vi "Reset1212(Host).vi"(2 "error in":errorcluster, 3 "FPGA Interface In":refnum<k20>) -> (0 "error out":errorcluster, 1 "FPGA Interface Out":refnum<k20>)   [LabVIEW 2018]
uses:
  <vilib>/userdefined/High Color/nirio_resource_hc.ctl
  <vilib>/FPGAPlugInAG/Dynamic/niLvFpga_Reset_Dynamic.vi
  <vilib>/Utility/error.llb/Error Cluster From Error Code.vi
  <vilib>/rvi/errors/niLvFpgaAdjustHostInterfaceError.vi
  <vilib>/FPGAPlugInAG/Dynamic/niLvFpga_Run_Dynamic.vi
  <vilib>/FPGAPlugInAG/Dynamic/niLvFpga_Close_Dynamic.vi
  <vilib>/rvi/interface/nirviMethod/nirviMethod.xnode
  <vilib>/rvi/interface/nirviReadWriteControl/nirviReadWriteControl.xnode
  <vilib>/rvi/interface/nirviCloseFPGA/nirviCloseFPGA.xnode
  NiFpgaLv.dll
  <vilib>/rvi/interface/Simulation/niFpgaSimulationCallBeginRW.vi
panel:
  in  "DEBUG":bool
  in  "resource name":T1="RIO0" caption="RIO Device"
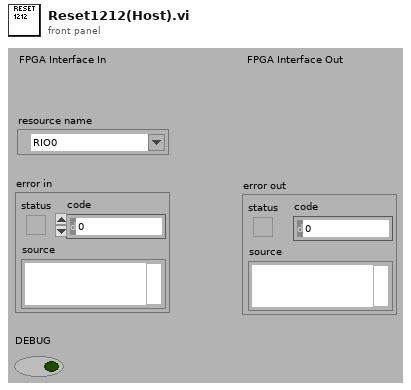
[diagram p1: front panel]
types:
  T1 = typedef "nirio_resource_hc.ctl" = tag
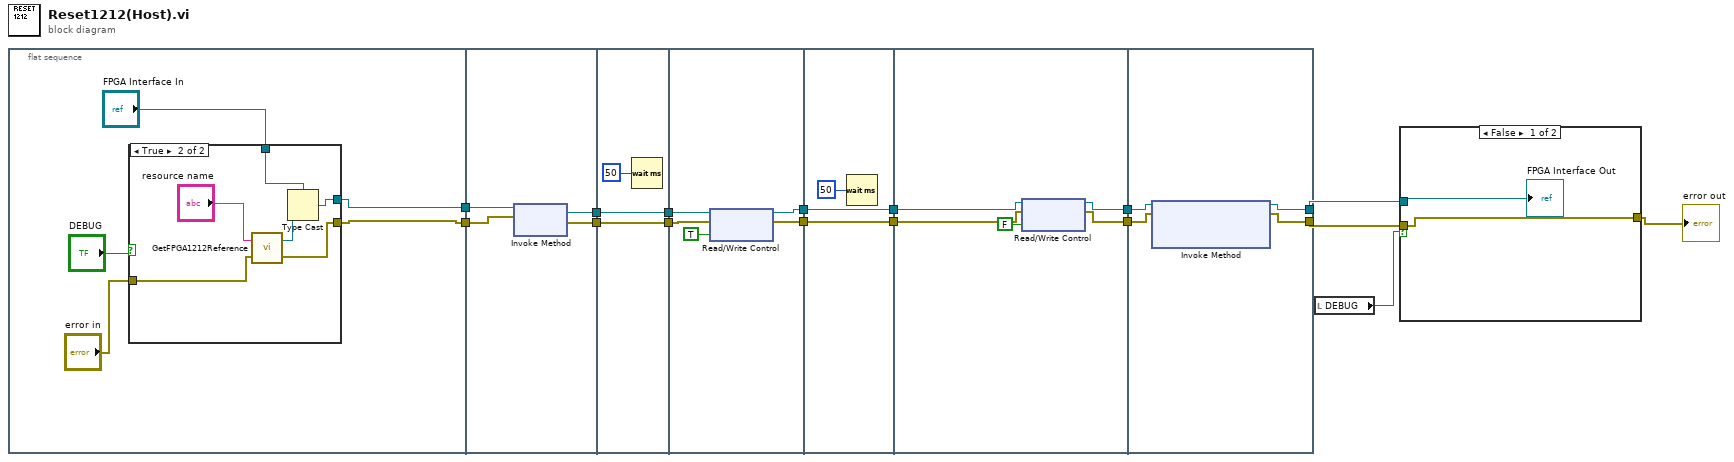
[diagram p0: block diagram]
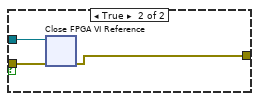
[diagram p2: hidden frame]
diagram:
  n1 = flat-sequence {
    tunnel: [w17] -> w9
    tunnel: [w18] -> w4
    tunnel: [w32] -> w8
    tunnel: w9 -> [w33]
    tunnel: [w31] -> w6
    tunnel: w4 -> [w30]
    tunnel: w8 -> [w36]
    tunnel: [w36] -> w7
    tunnel: w6 -> [w35]
    tunnel: [w35] -> w5
    tunnel: [w41] -> w16
    tunnel: [w40] -> w13
    tunnel: w7 -> [w37]
    tunnel: w5 -> [w38]
    tunnel: w16 -> [w43]
    tunnel: [w43] -> w15
    tunnel: [w42] -> w14
    tunnel: w13 -> [w42]
    tunnel: w15 -> [w49]
    tunnel: w14 -> [w48]
    tunnel: [w45] -> w3
    tunnel: [w46] -> w2
    tunnel: [w51] -> w11
    tunnel: [w50] -> w12
    tunnel: w3 -> [w52]
    tunnel: w2 -> [w53]
    frame #0 {
      n2 = case shown="True" "DEBUG" {
        tunnel: [w22 w28] -> w18
        tunnel: [w23 w25] -> w17
        tunnel: "error in" -> [w23 w26]
        tunnel: "FPGA Interface In" -> [w22 w29]
        frame False {
        }
        frame True {
          n3 = call "GetFPGA1212Reference.vi"("error in"=w26, "RIO Device IN"="resource name") -> ("error out"=w25:errorcluster, "FPGA VI Reference Out"=w24:refnum<k20>)
          n4 = Type Cast(type=w29, x=w24) -> (*(type *) &x=w28:refnum<k20>)
        }
      }
    }
    frame #1 {
      n5 = xnode "Invoke Method"("FPGA VI Reference In"=w30, "error in"=w33) -> ("FPGA VI Reference Out"=w32:refnum<k20>, "error out"=w31:errorcluster)
    }
    frame #2 {
      n6 = Wait (ms)(milliseconds to wait=u32 50) -> ()  [unwired: 1 out]
    }
    frame #3 {
      n7 = xnode "Read/Write Control"("FPGA VI Reference In"=w37, "error in"=w38, "SysReset"=TRUE ("WRITE MEM")) -> ("FPGA VI Reference Out"=w41:refnum<k20>, "error out"=w40:errorcluster)
    }
    frame #4 {
      n8 = Wait (ms)(milliseconds to wait=u32 50) -> ()  [unwired: 1 out]
    }
    frame #5 {
      n9 = xnode "Read/Write Control"("FPGA VI Reference In"=w49, "error in"=w48, "SysReset"=FALSE) -> ("FPGA VI Reference Out"=w46:refnum<k20>, "error out"=w45:errorcluster)
    }
    frame #6 {
      n10 = xnode "Invoke Method"("FPGA VI Reference In"=w53, "error in"=w52) -> ("FPGA VI Reference Out"=w51:refnum<k20>, "error out"=w50:errorcluster)  [unwired: 1 in]
    }
  }
  n11 = local read "DEBUG"() -> (w1:bool)
  n12 = case shown="False" w1 {
    tunnel: w12 -> [w55 w58]
    tunnel: w11 -> [w54 w57]
    tunnel: [w55 w56] -> w10
    frame False {
      "FPGA Interface Out" <- w54
    }
    frame True {
      n13 = xnode "Close FPGA VI Reference"("FPGA VI Reference In"=w57, "error in"=w58) -> ("error out"=w56:errorcluster)
    }
  }
  "error out" <- w10
